vi "Status Update.vi"(8 "error in (no error)":errorcluster, 10 "Status":string, 11 "Network Test in":refnum<class "Network Test.lvclass">) -> (0 "error out":errorcluster, 3 "Network Test out":refnum<class "Network Test.lvclass">)   [LabVIEW 2017, in "Network Test.lvlib" / "Network Test.lvclass"]
uses:
  Network Test.lvclass
  Network Test.lvclass/Network Test.ctl
  Test/Test/Test.lvclass
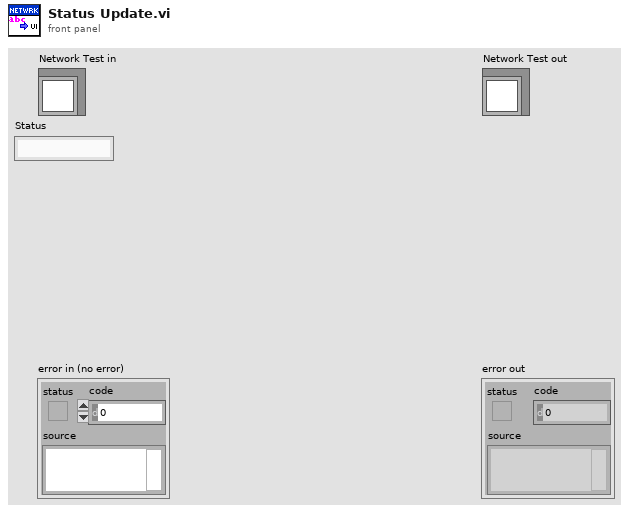
[diagram p1: front panel]
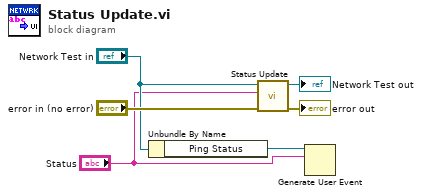
[diagram p0: block diagram]
diagram:
  n1 = Unbundle By Name("Network Test in") -> ("Ping Status"=w2:refnum<user-event>)
  n2 = call-parent "Status Update.vi"("error in (no error)"="error in (no error)", "Status"="Status", "Test in"="Network Test in") -> ("error out"=→"error out":errorcluster, "Test out"=→"Network Test out":refnum<class "Network Test.lvclass">)  [unwired: 7 in]
  n3 = Generate User Event(user event=w2, event data cluster="Status") -> ()  [unwired: 2 in, 2 out]
